vi "Read Local Resource.vi"(8 "error in (no error)":errorcluster, 11 "SimELoad in":refnum<class "SimEload.lvclass">) -> (0 "error out":errorcluster, 2 "Local Resource":refnum<visa-resource-name>, 3 "SimELoad out":refnum<class "SimEload.lvclass">)   [LabVIEW 2019, in "SimELoad.lvlib" / "SimEload.lvclass"]
uses:
  SimEload.lvclass
  SimEload.lvclass/SimEload.ctl
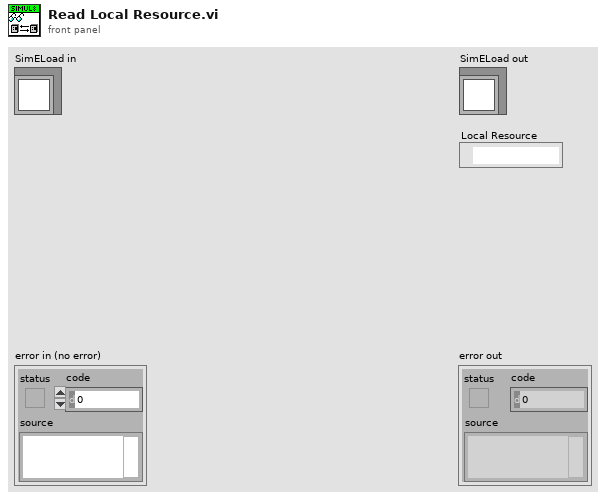
[diagram p1: front panel]
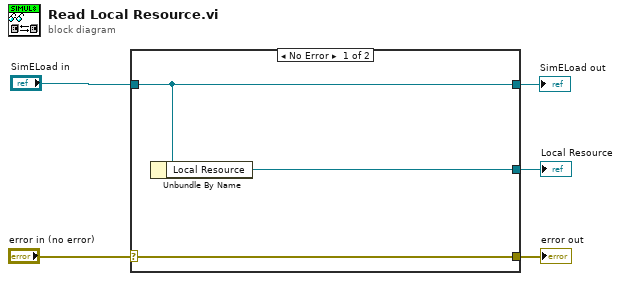
[diagram p0: block diagram]
diagram:
  n1 = case shown="No Error" "error in (no error)" {
    selector: "error in (no error)" -> [w8 w9]
    tunnel: [w8 w9] -> w4
    tunnel: [w7 w10] -> w3
    tunnel: "SimELoad in" -> [w7 w10]
    tunnel: [w6 _] -> w2
    frame No Error {
      n2 = Unbundle By Name(w7) -> ("Local Resource"=w6:refnum<visa-resource-name>)
    }
    frame Error {
    }
  }
  "error out" <- w4
  "Local Resource" <- w2
  "SimELoad out" <- w3
